vi "getrealandimagejob.vi"(0 "sample port":refnum<visa-resource-name>[](array[refnum]), 2 "sample sn":string[](array[string]), 5 "isred":bool) -> (4 "error":errorcluster[](array[cluster]), 6 "real":dbl[](array[numeric]), 7 "Array":bool[](array[boolean]), 8 "image":dbl[](array[numeric]))   [LabVIEW 2012]
uses:
  globalstatus.vi
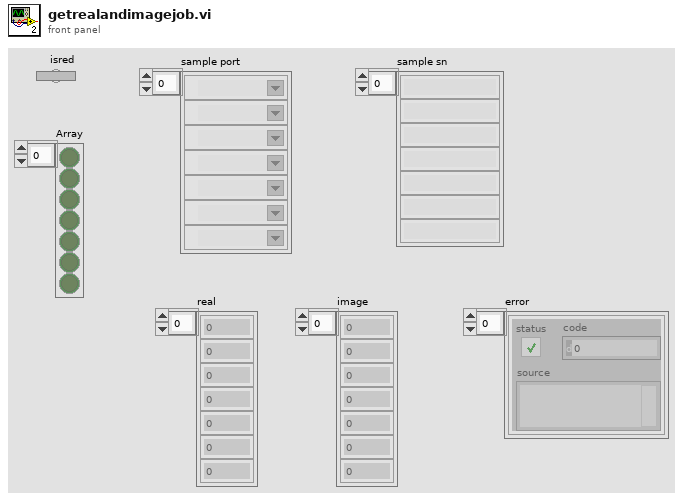
[diagram p1: front panel]
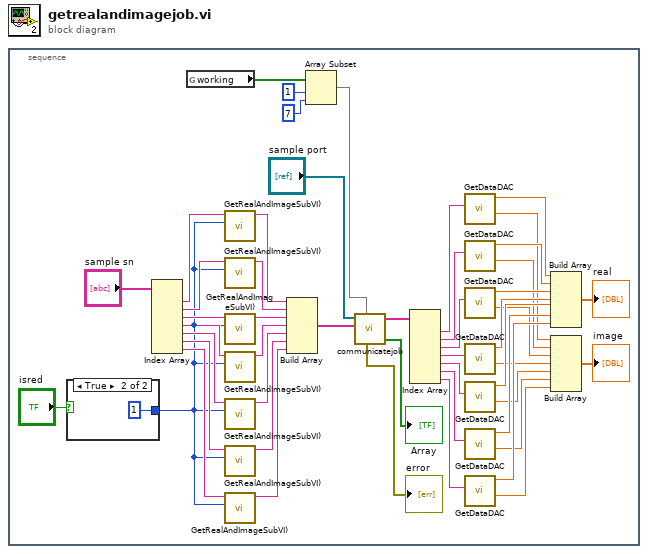
[diagram p0: block diagram]
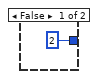
[diagram p2: hidden frame]
diagram:
  n1 = stacked-sequence {
    frame #0 {
      n2 = case shown="True" "isred" {
        tunnel: [2 1] -> w40
        frame False {
        }
        frame True {
        }
      }
      n3 = Index Array(array="sample sn") -> (element #1=w41:string, element #2=w42:string, element #3=w43:string, element #4=w44:string, element #5=w45:string, element #6=w46:string, element #7=w47:string)  [unwired: 7 in]
      n4 = global read "globalstatus.vi" "working"() -> (w3:bool[])
      n5 = call "GetRealAndImageSubVI).vi"("byte data"=w40, "sn"=w41) -> ("output frame"=w12:string)  [unwired: 9 in]
      n6 = call "GetRealAndImageSubVI).vi"("byte data"=w40, "sn"=w42) -> ("output frame"=w11:string)  [unwired: 9 in]
      n7 = call "GetRealAndImageSubVI).vi"("byte data"=w40, "sn"=w43) -> ("output frame"=w10:string)  [unwired: 9 in]
      n8 = call "GetRealAndImageSubVI).vi"("byte data"=w40, "sn"=w44) -> ("output frame"=w9:string)  [unwired: 9 in]
      n9 = call "GetRealAndImageSubVI).vi"("byte data"=w40, "sn"=w45) -> ("output frame"=w8:string)  [unwired: 9 in]
      n10 = call "GetRealAndImageSubVI).vi"("byte data"=w40, "sn"=w46) -> ("output frame"=w7:string)  [unwired: 9 in]
      n11 = call "GetRealAndImageSubVI).vi"("byte data"=w40, "sn"=w47) -> ("output frame"=w6:string)  [unwired: 9 in]
      n12 = Build Array(w12, w11, w10, w9, w8, w7, w6) -> (w13:string[])
      n13 = Array Subset(array=w3, index=1, length=7) -> (w4:bool[])
      n14 = call "communicatejob.vi"("sample port"="sample port", "condition"=w4, "send command"=w13) -> ("error"=→"error":errorcluster[], "receive data"=w23:string[], "receive result"=→"Array":bool[])  [unwired: 2 in, 1 out]
      n15 = Index Array(array=w23) -> (element #1=w21:string, element #2=w20:string, element #3=w19:string, element #4=w18:string, element #5=w17:string, element #6=w16:string, element #7=w15:string)  [unwired: 7 in]
      n16 = call "GetDataDAC.vi"("data"=w21) -> ("blue"=w26:dbl, "red"=w39:dbl)  [unwired: 9 in]
      n17 = call "GetDataDAC.vi"("data"=w20) -> ("blue"=w27:dbl, "red"=w38:dbl)  [unwired: 9 in]
      n18 = call "GetDataDAC.vi"("data"=w19) -> ("blue"=w28:dbl, "red"=w37:dbl)  [unwired: 9 in]
      n19 = call "GetDataDAC.vi"("data"=w18) -> ("blue"=w29:dbl, "red"=w36:dbl)  [unwired: 9 in]
      n20 = call "GetDataDAC.vi"("data"=w17) -> ("blue"=w30:dbl, "red"=w35:dbl)  [unwired: 9 in]
      n21 = call "GetDataDAC.vi"("data"=w16) -> ("blue"=w31:dbl, "red"=w34:dbl)  [unwired: 9 in]
      n22 = call "GetDataDAC.vi"("data"=w15) -> ("blue"=w32:dbl, "red"=w33:dbl)  [unwired: 9 in]
      n23 = Build Array(w39, w38, w37, w36, w35, w34, w33) -> (→"real":dbl[])
      n24 = Build Array(w26, w27, w28, w29, w30, w31, w32) -> (→"image":dbl[])
    }
  }
